vi "Global Angle.vi"() -> ()   [LabVIEW 2015]
panel:
  in  "Kill":bool
  in  "Mode":enum16{"Normal", "Zero", "Kinamatic", "Camera"}(ring)
  out "Current Wrist":dbl(slide) scale=-100.0..100.0
  out "Current Shoulder":dbl(slide) scale=-40.0..33.0
  out "WristStop":bool
  out "WristBusy":bool
  out "ShoulderStop":bool
  out "ShoulderBusy":bool
  in  "Grip":bool
  in  "PiceAngle":dbl(slide) scale=0.0..180.0
  in  "GripperAngle":dbl(slide) scale=-20.0..100.0
  out "startedWristBit":bool
  in  "Wrist integral":dbl
  in  "Wrist Angle":dbl(slide) scale=-100.0..100.0
  in  "Shoulder Angle":dbl(slide) scale=-40.0..33.0
  # "Wrist"
  # "Shoulder"
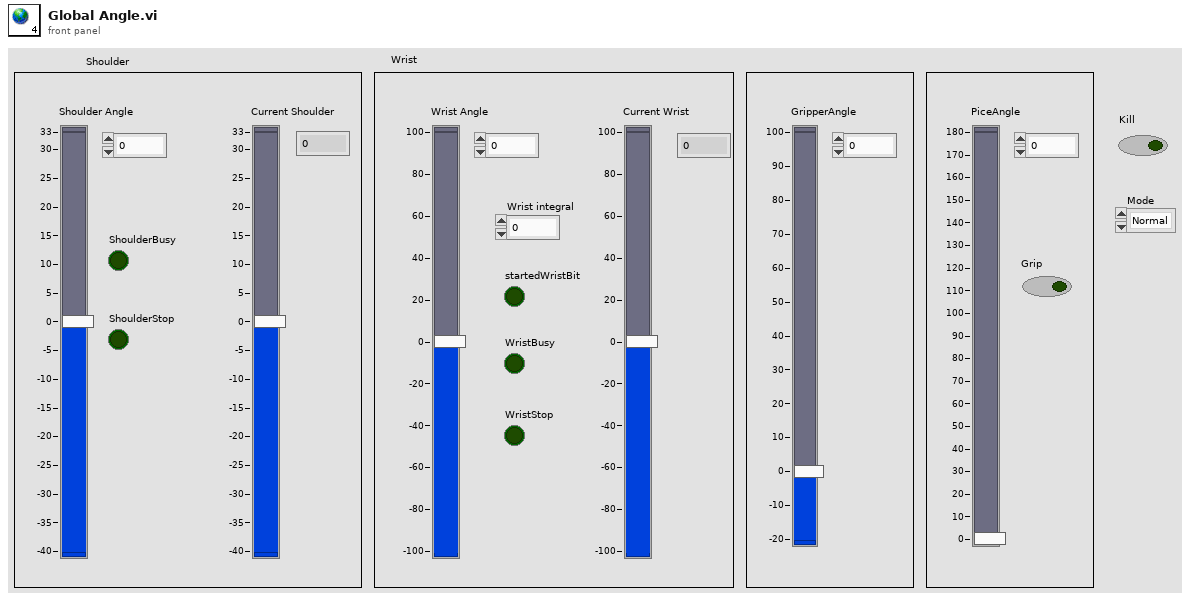
[diagram p1: front panel]
diagram:
